vi "Final G bak.vi"() -> ()   [LabVIEW 2014]
uses:
  <vilib>/Instr/_visa.llb/VISA Configure Serial Port (Instr).vi
panel:
  out "read buffer":string
  in  "Threshold":string
  in  "Password":string
  out "return count read":u32
  in  "VISA resource name":refnum<visa-resource-name>
  out "password is wrong":bool
  in  "stop":bool
  out "Iteration":i32
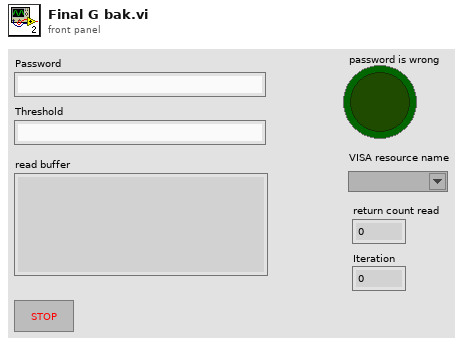
[diagram p1: front panel]
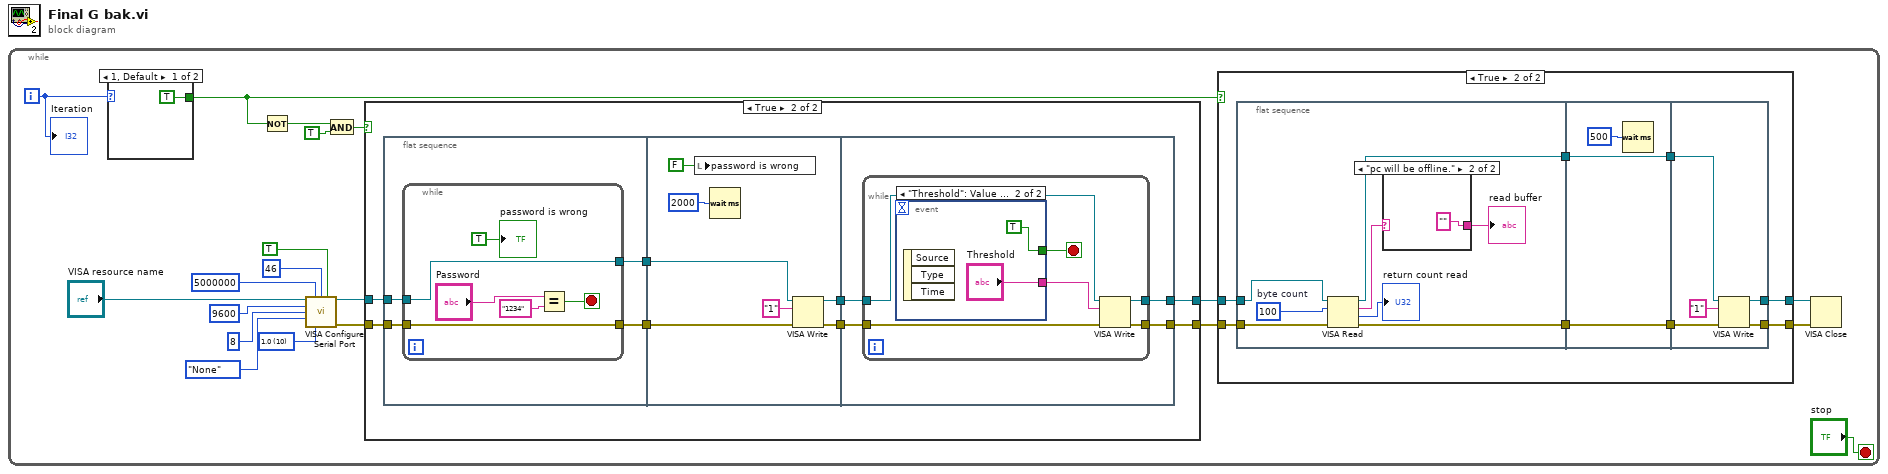
[diagram p0: block diagram]
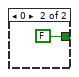
[diagram p2: hidden frame]
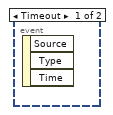
[diagram p6: hidden frame]
diagram:
  n1 = while {
    i -> [w3]
    stop <- "stop" stop-if-true
    w17 = u16 10 items=["1.0"=10, "1.5"=15, "2.0"=20] ("stop bits (10: 1 bit)")
    n2 = case shown="1, Default" w3 {
      tunnel: [TRUE FALSE] -> w2
      frame 1, Default {
      }
      frame 0 {
      }
    }
    n3 = Not(x=w2) -> (.not. x?=w12:bool)
    n4 = call-poly "VISA Configure Serial Port"("VISA resource name"="VISA resource name", "timeout (10sec)"=u32 5000000, "termination char\n(0xA = '\\n' = LF)"=u8 46 ("termination char\n(0xA = '\\n' = LF)"), "Enable Termination\nChar (T)"=TRUE ("Enable Termination\nChar (T)"), "baud rate (9600)"=u32 9600, "data bits (8)"=u16 8, "parity (0:none)"=enum16{"None", "Odd", "Even", "Mark", "Space"}."None", "stop bits (10: 1 bit)"=w17) -> ("VISA resource name out"=w11:refnum<visa-resource-name>, "error out"=w10:errorcluster)  [unwired: 6 in]
    n5 = And(x=w12, y=TRUE) -> (x .and. y?=w9:bool)
    n6 = case shown="True" w9 {
      tunnel: w10 -> [w52 w60]
      tunnel: [w51 w58] -> w8
      tunnel: [w52 w57] -> w6
      tunnel: w11 -> [w51 w59]
      frame False {
      }
      frame True {
        n7 = flat-sequence {
          tunnel: w60 -> [w64]
          tunnel: w59 -> [w63]
          tunnel: [w62] -> w56
          tunnel: [w61] -> w55
          tunnel: w56 -> [w77]
          tunnel: w55 -> [w76]
          tunnel: [w75] -> w54
          tunnel: [w74] -> w53
          tunnel: [w80] -> w58
          tunnel: [w79] -> w57
          tunnel: w54 -> [w81]
          tunnel: w53 -> [w78]
          frame #0 {
            n8 = while {
              tunnel: w64 -> [w68]
              tunnel: w63 -> [w67]
              tunnel: [w68] -> w62
              tunnel: [w67] -> w61
              stop <- w69 stop-if-true
              n9 = Equal?(x="Password", y="1234") -> (x = y?=w69:bool)
              "password is wrong" <- TRUE
            }
          }
          frame #1 {
            n10 = local write "password is wrong"(FALSE) -> ()
            n11 = Wait (ms)(milliseconds to wait=u32 2000) -> ()  [unwired: 1 out]
            n12 = VISA Write(VISA resource name=w76, write buffer="1", error in (no error)=w77) -> (VISA resource name out=w75:refnum<visa-resource-name>, error out=w74:errorcluster)  [unwired: 1 out]
          }
          frame #2 {
            n13 = while {
              tunnel: w81 -> [w87]
              tunnel: [w86] -> w80
              tunnel: [w85] -> w79
              tunnel: w78 -> [w84]
              stop <- w83 stop-if-true
              n14 = event shown="[1] \"Threshold\": Value Change" {
                selector: _ -> [_ _]
                dyn-events: _ -> [_ _]
                timeout: _ -> [_ _]
                tunnel: [_ TRUE] -> w83
                tunnel: [_ "Threshold"] -> w82
                event Timeout {
                  n15 = event-data() -> ()  [unwired: 1 in, 3 out]
                }
                event "Threshold": Value Change {
                  n16 = event-data() -> ()  [unwired: 1 in, 3 out]
                }
              }
              n17 = VISA Write(VISA resource name=w87, write buffer=w82, error in (no error)=w84) -> (VISA resource name out=w86:refnum<visa-resource-name>, error out=w85:errorcluster)  [unwired: 1 out]
            }
          }
        }
      }
    }
    n18 = case shown="True" w2 {
      tunnel: [w24 w30] -> w7
      tunnel: [w23 w32] -> w5
      tunnel: w8 -> [w24 w31]
      tunnel: w6 -> [w23 w25]
      frame False {
      }
      frame True {
        n19 = flat-sequence {
          tunnel: w31 -> [w38]
          tunnel: [w40] -> w29
          tunnel: [w37] -> w27
          tunnel: w25 -> [w36]
          tunnel: w29 -> [w45]
          tunnel: [w45] -> w28
          tunnel: w27 -> [w44]
          tunnel: [w44] -> w26
          tunnel: [w47] -> w30
          tunnel: [w46] -> w32
          tunnel: w28 -> [w48]
          tunnel: w26 -> [w49]
          frame #0 {
            w35 = u32 100  # byte count
            n20 = VISA Read(VISA resource name=w38, byte count=w35, error in (no error)=w36) -> (VISA resource name out=w37:refnum<visa-resource-name>, read buffer=w34:string, return count=→"return count read":u32, error out=w40:errorcluster)
            n21 = case shown="\"pc will be offline.\"" w34 {
              selector: w34 -> [w41 _]
              tunnel: [w41 ""] -> w33
              frame "False", Default {
              }
              frame "pc will be offline." {
              }
            }
            "read buffer" <- w33
          }
          frame #1 {
            n22 = Wait (ms)(milliseconds to wait=u32 500) -> ()  [unwired: 1 out]
          }
          frame #2 {
            n23 = VISA Write(VISA resource name=w49, write buffer="1", error in (no error)=w48) -> (VISA resource name out=w47:refnum<visa-resource-name>, error out=w46:errorcluster)  [unwired: 1 out]
          }
        }
      }
    }
    n24 = VISA Close(VISA resource name=w7, error in (no error)=w5) -> ()  [unwired: 1 out]
    "Iteration" <- w3
  }
